vi "SDT_DecompressData.vi"(8 "ErrorIn":errorcluster, 11 "CompressedData":u8[](array[numeric])) -> (0 "ErrorOut":errorcluster, 3 "DecompressedData(U16)":u16[](array[numeric]))   [LabVIEW 2019]
doc: "Use this VI to decompress ZIPped data blocks in SDT-files. We utilize LV's own Unzip.vi but need to write the data block to disc for that.\nSpecial care needs to be taken not to decompress the data into an array larger than x8000 0000 = d2.147.483.648 which is the LV array's largest index value. (I32)\n\ninfo@becker-hickl.com"
uses:
  <vilib>/zip/NI_Unzip.lvlib
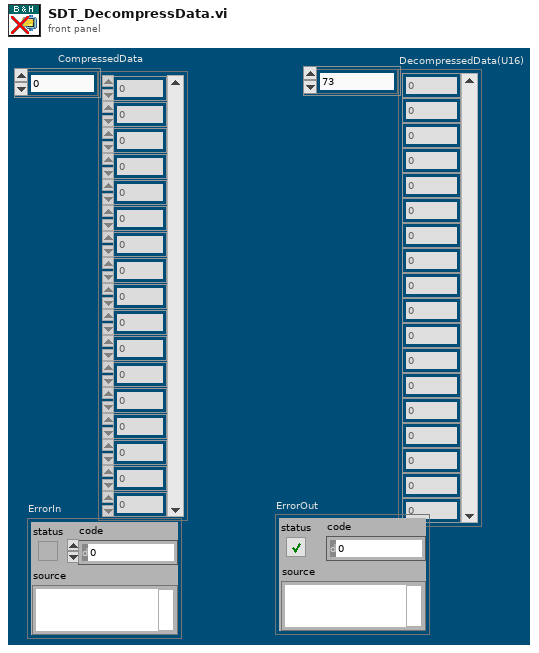
[diagram p1: front panel]
types:
  T1 = enum16{"big-endian, network order", "native, host order", "little-endian"}
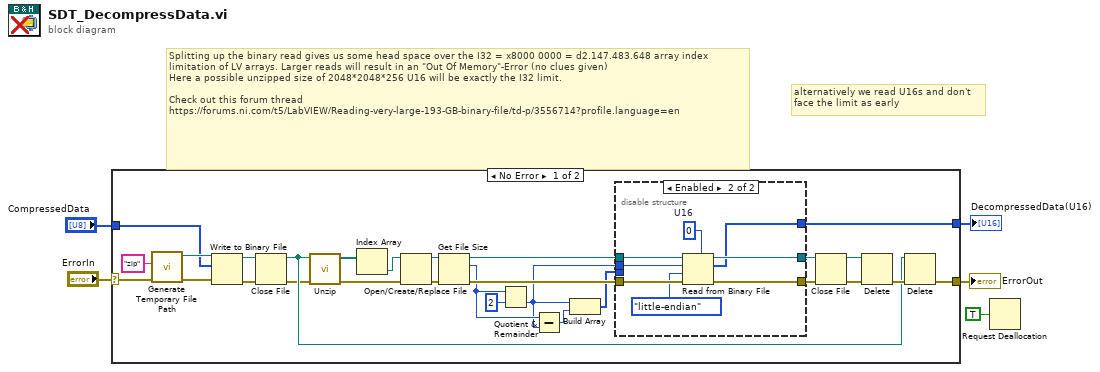
[diagram p0: block diagram]
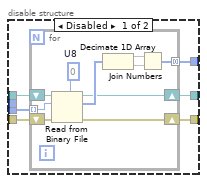
[diagram p2: hidden frame]
diagram:
  # "alternatively we read U16s and don't\nface the limit as early"
  # "Splitting up the binary read gives us some head space over the I32 = x8000 0000 = d2.147.483.648 array index\nlimitation of LV arrays. Larger reads will result in an \"Out Of Memory\"-Error (no clues given) \nHere a possible unzipped size of 2048*2048*256 U16 will be exactly the I32 limit.\n\nCheck out this forum thread\nhttps://forums.ni.com/t5/LabVIEW/Reading-very-large-193-GB-binary-file/td-p/3556714?profile.language=en"
  n1 = case shown="No Error" "ErrorIn" {
    selector: "ErrorIn" -> [w31 w58]
    tunnel: [w33 _] -> w5
    tunnel: [w27 w58] -> w3
    tunnel: "CompressedData" -> [w21 _]
    frame No Error {
      n2 = call <vilib>:"Generate Temporary File Path.vi"("error in (no error)"=w31, "Temporary File Extension (tmp)"="zip" ("time format string (%c)")) -> ("error out"=w25:errorcluster, "Unique Temporary File Path"=w26:path)  [unwired: 8 in]
      n3 = Write to Binary File(file (use dialog)=w26, data=w21, error in=w25) -> (refnum out=w19:refnum<file>, error out=w17:errorcluster)  [unwired: 3 in, 1 out]
      n4 = Close File(refnum=w19, error in=w17) -> (path=w22:path, error out=w18:errorcluster)
      n5 = call <vilib>:"Unzip.vi"("error in (no error)"=w18, "Zip file"=w22) -> ("error out"=w15:errorcluster, "Unzipped files"=w20:path[])  [unwired: 7 in, 1 out]
      n6 = Index Array(array=w20) -> (element=w16:path)  [unwired: 1 in]
      n7 = Open/Create/Replace File(file path (use dialog)=w16, error in=w15) -> (refnum out=w11:refnum<file>, error out=w12:errorcluster)  [unwired: 4 in, 1 out]
      n8 = Get File Size(file=w11, error in=w12) -> (refnum out=w9:refnum<file>, size (in bytes)=w7:i64, 0:w10:errorcluster)
      n9 = Quotient & Remainder(x=w7, y=i64 2) -> (floor(x/y)=w6:i64)  [unwired: 1 out]
      n10 = Subtract(x=w7, y=w6) -> (x-y=w14:i64)
      n11 = Build Array(w6, w14) -> (w8:i64[])
      n12 = disable-structure shown="Enabled" {
        disable-tunnel: [w39 w51] -> w33
        disable-tunnel: [w38 w57] -> w24
        disable-tunnel: [w37 w56] -> w23
        disable-tunnel: w10 -> [w36 w55]
        disable-tunnel: w9 -> [w35 w54]
        disable-tunnel: w8 -> [w34 _]
        disable-tunnel: w6 -> [_ w52]
        frame Disabled {
          n13 = for {
            tunnel: [w49] -> w39 mode=concatenating
            shift-right: [w47] -> w38
            shift-left: w36 -> [w42]
            shift-right: [w46] -> w37
            shift-left: w35 -> [w41]
            tunnel: w34 -> [w40] mode=indexing
            w45 = u8 0  # U8
            n14 = Read from Binary File(5:w45, 8:w42, 10:w40, 11:w41) -> (0:w47:errorcluster, 2:w48:u8[], 3:w46:refnum<file>)  [unwired: 2 in, 1 out]
            n15 = Decimate 1D Array(w48) -> (w44:u8[], w43:u8[])
            n16 = Join Numbers(hi=w44, lo=w43) -> ((hi.lo)=w49:u16[])
          }
        }
        frame Enabled {
          w53 = u16 0  # U16
          n17 = Read from Binary File(5:w53, 8:w55, 9:T1."little-endian" ("byte order (0:big-endian, network order)"), 10:w52, 11:w54) -> (0:w57:errorcluster, 2:w51:u16[], 3:w56:refnum<file>)  [unwired: 1 in, 1 out]
        }
      }
      n18 = Close File(refnum=w23, error in=w24) -> (path=w28:path, error out=w30:errorcluster)
      n19 = Delete(path (use dialog)=w28, error in=w30) -> (error out=w29:errorcluster)  [unwired: 3 in, 2 out]
      n20 = Delete(path (use dialog)=w22, error in=w29) -> (error out=w27:errorcluster)  [unwired: 3 in, 2 out]
    }
    frame Error {
    }
  }
  "DecompressedData(U16)" <- w5
  "ErrorOut" <- w3
  n21 = Request Deallocation(TRUE ("flag")) -> ()
